vi "Bring Window to Front.vi"() -> ()   [LabVIEW 2023]
uses:
  User32.dll
panel:
  in  "stop":bool
  in  "Window Name":string
  in  "Go":bool
  out "Handle":u64
  out "Error":i32
  out "error out":errorcluster
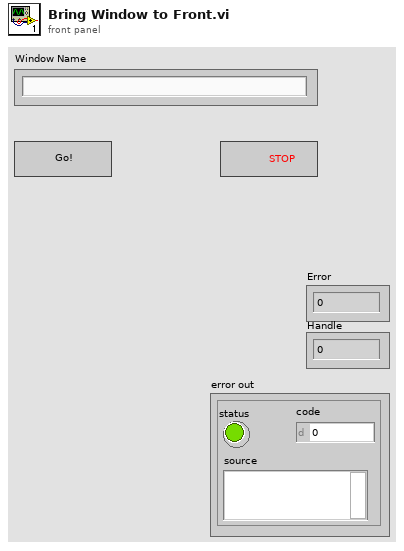
[diagram p1: front panel]
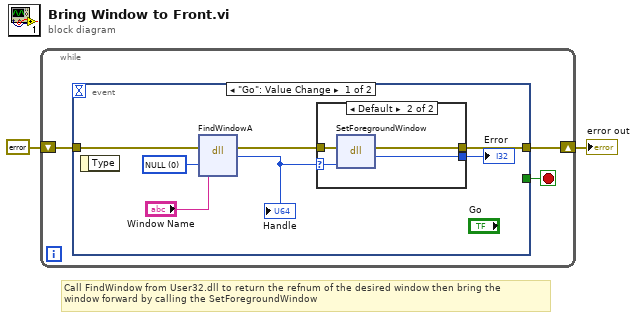
[diagram p0: block diagram]
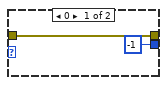
[diagram p2: hidden frame]
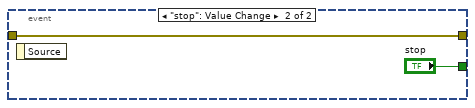
[diagram p3: hidden frame]
diagram:
  # "Call FindWindow from User32.dll to return the refnum of the desired window then bring the \nwindow forward by calling the SetForegroundWindow"
  n1 = while {
    shift-right: [w4] -> w2
    shift-left: errorcluster {"status"=FALSE, "code"=0, "source"=""} ("error out") -> [w3]
    stop <- w5 stop-if-true
    n2 = event shown="[0] \"Go\": Value Change" {
      selector: _ -> [_ _]
      dyn-events: _ -> [_ _]
      timeout: _ -> [_ _]
      tunnel: [_ "stop"] -> w5
      tunnel: [w8 w19] -> w4
      tunnel: w3 -> [w7 w19]
      event "Go": Value Change {
        w12 = 0 items=["NULL"]
        n3 = event-data() -> ()  [unwired: 2 out]
        n4 = dll-call lib="user32.dll" fn="FindWindowA" label="FindWindow"(error in=w7, "lpszClassName"=w12, "lpszWindowName"="Window Name") -> (error out=w9:errorcluster, "hWnd"=w6:u64)  [unwired: 3 in, 2 out]
        "Handle" <- w6
        n5 = case shown="Default" w6 {
          selector: w6 -> [_ w15]
          tunnel: [-1 ("return type") w18] -> w10
          tunnel: w9 -> [w14 w17]
          tunnel: [w14 w16] -> w8
          frame 0 {
          }
          frame Default {
            n6 = dll-call lib="user32.dll" fn="SetForegroundWindow"(error in=w17, "Handle"=w15) -> (error out=w16:errorcluster, "return type"=w18:i32)  [unwired: 3 in, 1 out]
          }
        }
        "Error" <- w10
      }
      event "stop": Value Change {
        n7 = event-data() -> ()  [unwired: 2 out]
      }
    }
  }
  "error out" <- w2
